vi "SetBrokerParam.vi"(6 "Enum":enum16{"Remote", "Local"}(ring), 7 "error in":errorcluster, 8 "ParamVAL":i32, 9 "ParamIDX":T1(ring)=enum."TCP/UDP Port", 10 "DeviceID":u8=1, 11 "Handle In":u64[](array[numeric])) -> (2 "Result":i32, 3 "Handle Out":u64[](array[numeric]), 5 "error out":errorcluster)   [LabVIEW 2020, in "SnapMB.lvlib"]
uses:
  SnapMB.lvlib
  windows/snapmb.dll
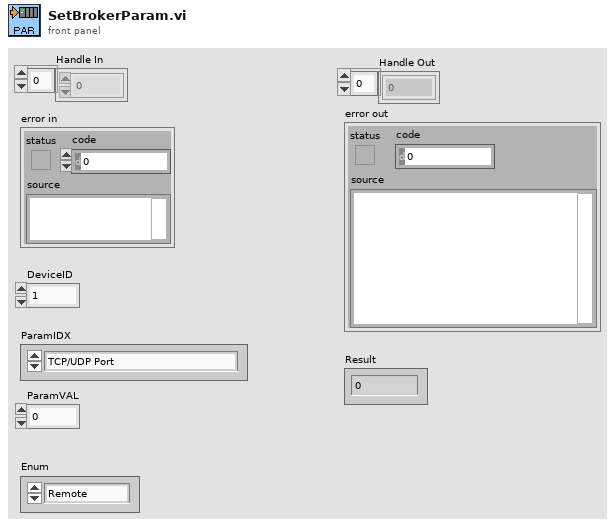
[diagram p1: front panel]
types:
  T1 = enum16{"No Param", "TCP/UDP Port", "DeviceID", "TCP Persistence", "Disconnect On Error", "Send Timeout", "Serial Format", "Auto Timeout", "Auto Time Limit Min", "Fixed Timeout", "Base Address", "Is Gateway", "Peer List Mode", "Packet Log", "Interframe Delay", "Work Interval", "Allow Serial Functions on Ethernet", "Max Retries", "Disconnect Timeout", "Attempt Sleep"}
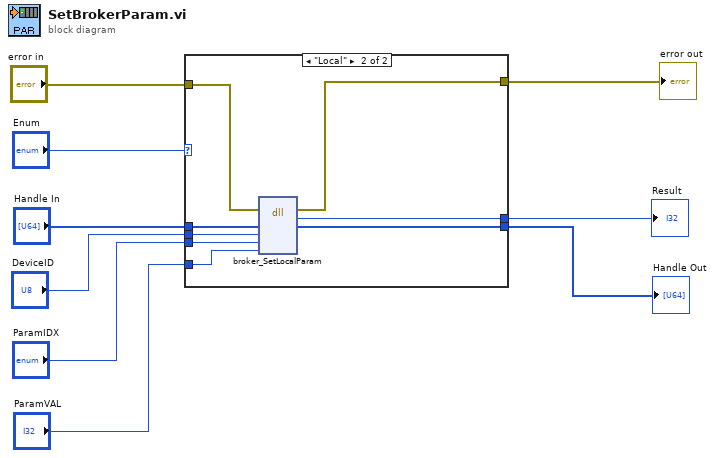
[diagram p0: block diagram]
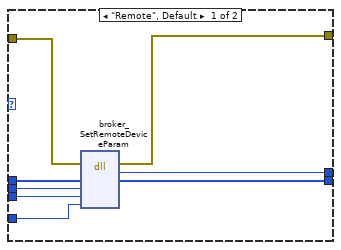
[diagram p2: hidden frame]
diagram:
  n1 = case shown="\"Local\"" "Enum" {
    tunnel: "Handle In" -> [w16 w25]
    tunnel: [w10 w24] -> w8
    tunnel: [w12 w23] -> w7
    tunnel: "error in" -> [w17 w22]
    tunnel: "DeviceID" -> [w15 w21]
    tunnel: "ParamVAL" -> [w13 w20]
    tunnel: [w11 w19] -> w3
    tunnel: "ParamIDX" -> [w14 w18]
    frame "Remote", Default {
      n2 = dll-call lib="D:/SnapMB/LabVIEW/lib/windows/snapmb.dll" fn="broker_SetRemoteDeviceParam"(error in=w17, "Broker"=w16, "DeviceID"=w15, "ParamIDX"=w14, "ParamVAL"=w13) -> (error out=w12:errorcluster, "Result"=w11:i32, "Broker"=w10:u64[])  [unwired: 5 in, 1 out]
    }
    frame "Local" {
      n3 = dll-call lib="D:/SnapMB/LabVIEW/lib/windows/snapmb.dll" fn="broker_SetLocalParam"(error in=w22, "Broker"=w25, "DeviceID"=w21, "ParamIDX"=w18, "ParamVAL"=w20) -> (error out=w23:errorcluster, "Result"=w19:i32, "Broker"=w24:u64[])  [unwired: 5 in, 1 out]
    }
  }
  "Handle Out" <- w8
  "error out" <- w7
  "Result" <- w3
